vi "Take Registry Ownership.vi"(9 "Registry Configuration (Init only)":T1, 10 "Initialize (F)":bool, 11 "Token":string) -> ()   [LabVIEW 2014, in "UniqueName.lvlib" / "UniqueName.lvclass"]
uses:
  UniqueName.lvclass
  RegistryConfiguration.ctl
  Delimiter/Delimiter.lvclass
  RandomStringGenerator/RandomStringGenerator.lvclass
  UniquenessCriteria/UniquenessCriteria.lvclass
  Command.ctl
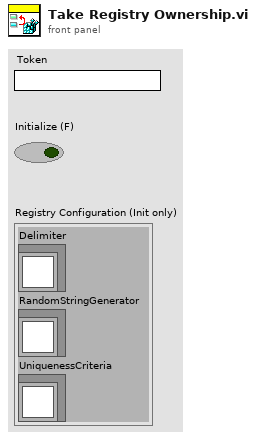
[diagram p1: front panel]
types:
  T1 = typedef "UniqueName.lvlib/UniqueName.lvclass/RegistryConfiguration.ctl" = cluster{"Delimiter":refnum<class "Delimiter.lvclass">, "RandomStringGenerator":refnum<class "RandomStringGenerator.lvclass">, "UniquenessCriteria":refnum<class "UniquenessCriteria.lvclass">}
  T2 = typedef "UniqueName.lvlib/UniqueName.lvclass/Command.ctl" = enum16{"Get", "Get All", "Set", "Delete", "Get Status", "Init", "Reserve Ownership", "Release Ownership", "Lock", "Unlock"}
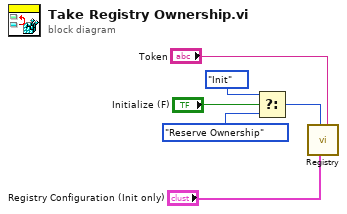
[diagram p0: block diagram]
diagram:
  n1 = Select(t=Command."Init" ("Command (Get)"), s="Initialize (F)", f=Command."Reserve Ownership" ("Command (Get)")) -> (s? t:f=w3:T2)
  n2 = call "Registry.vi"("Token"="Token", "Registry Configuration"="Registry Configuration (Init only)", "Command (Get)"=w3) -> ()  [unwired: 4 in, 5 out]
